vi "Init.vi"() -> (3 "Queue Transport out":refnum<class "Queue Transport.lvclass">)   [LabVIEW 2025, in "jettl.lvlib" / "Transport.lvlib" / "Queue Transport.lvclass"]
uses:
  Queue Transport.lvclass
  Queue Transport.lvclass/Queue Transport.ctl
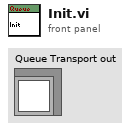
[diagram p1: front panel]
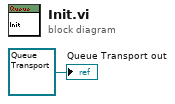
[diagram p0: block diagram]
diagram:
  "Queue Transport out" <- refnum<class "Queue Transport.lvclass"> refnum ("Queue Transport out")
